vi "e.gate Example - ASCII Write Value.vi"() -> ()   [LabVIEW 2016]
doc: "<B>AMC - Analytik & Messtechnik GmbH Chemnitz</B>\n\nLabVIEW Drivers for e.gate / e.pac series from Gantner Instruments\n\nThis VI demonstrates the usage of the driver by writing an analog value to the e.gate/e.pac device."
uses:
  e.gate Protocol Type.ctl
  e.gate ASCII Write Value - Integer.vi
panel:
  in  "Value":i32
  in  "IP Address":string="10.0.10.54"
  in  "Channel":i32
  in  "stop":bool
  out "error out":errorcluster
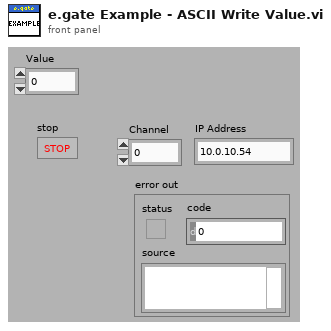
[diagram p1: front panel]
types:
  T1 = typedef "e.gate Protocol Type.ctl" = enum16{"ASCII", "HighspeedPort Online", "HighspeedPort Buffer", "eGateHighspeedPortDLL "}
  T2 = typedef "e.gate Configuration.ctl" = cluster{"connection ID":refnum<k5>, "IPAddress":string, "BufferIndex":i32, "StateMessage":string, "StateCode":i8, "HeaderSize":i32, "BufferSize":i32, "IsBigEndian":i32, "Version":i32, "ChannelCount":i32, "FrameLength":i32, "StartTime":dbl, "dActTimeToSecondFactor":dbl, "StartTimeToDayFactor":dbl, "BufferFillRate":dbl, "SampleRate":dbl, "ChannelData":T3[], "DecodeTimeFormat":string, "SummaryPath":string, "WithCheckSum":i32, "dActTimeDataType":T4, "MaxWriteCount":i32, "MaxReadCount":i32, "TempOffsetRead":i32, "TempLengthRead":i32, "Protocol":T1, "IsSupported":i32, "InputAccessList":i32[], "OutputAccessList":i32[], "DataSource":enum16{"CircleBuffer", "test.con Logger", "test.con Archive"}, "Modules":T5[], "DLL-Handle":T6}
  T3 = typedef "e.gate Channel Data.ctl" = cluster{"VariableName":string, "DataDirection":string, "DataType":string, "DataTypeIndex":T4, "Precision":i16, "FieldLengtht":i16, "ByteCount":i32, "Format":string, "Unit":string, "InputAccessOffset":i32, "OutputAccessOffset":i16, "InputAccessIndex":i16, "OutputAccessIndex":i16, "VarType":string}
  T4 = typedef "e.gate Data Type.ctl" = enum16{"NO", "BOOL", "SINT8", "USINT8", "SINT16", "USINT16", "SINT32", "USINT32", "FLOAT", "SET8", "SET16", "SET32", "DOUBLE", "SINT64", "USINT64", "SET64"}
  T5 = typedef "e.gate Module  Data.ctl" = cluster{"Type":string, "Location":string, "VariablesCount":i16, "UartIndex":i16, "Address":i16, "SystemOffset":i16}
  T6 = typedef "e.gateHSP_DLLhandle.ctl" = cluster{"clientInstance":i32, "connectionInstance":i32}
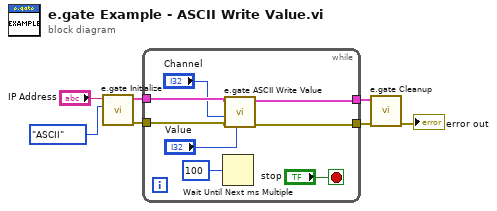
[diagram p0: block diagram]
diagram:
  n1 = call "e.gate Initialize.vi"("Protocol"=e.gate_Protocol_Type."ASCII", "IP Address"="IP Address") -> ("error out"=w3:errorcluster, "e.gate Configuration"=w2:T2)  [unwired: 8 in]
  n2 = while {
    tunnel: [w12] -> w5
    tunnel: [w13] -> w4
    tunnel: w3 -> [w9]
    tunnel: w2 -> [w11]
    stop <- "stop" stop-if-true
    n3 = Wait Until Next ms Multiple(millisecond multiple=u32 100) -> ()  [unwired: 1 out]
    n4 = call-poly "e.gate ASCII Write Value.vi"("Value"="Value", "error in (no error)"=w9, "Channel"="Channel", "e.gate Configuration In"=w11) -> ("error out"=w12:errorcluster, "e.gate Configuration Out"=w13:T2)  [unwired: 6 in]
  }
  n5 = call "e.gate Cleanup.vi"("error in (no error)"=w5, "e.gate Configuration"=w4) -> ("error out"=→"error out":errorcluster)  [unwired: 9 in]
